vi "BC Verify Minor Frame Subroutine.vi"(5 "Instruction ID":i32, 6 "Pointers":T1={"Major Command Pointer"=2206, "Major Data Pointer"=2206, "Minor Command Pointer"=2206, "Minor Data Pointer"=2206}, 7 "Target IC (1-8)":u8, 8 "error in (no error)":errorcluster, 11 "Bus Controller in":refnum<class "Bus Controller.lvclass">) -> (0 "error out":errorcluster, 3 "Bus Controller out":refnum<class "Bus Controller.lvclass">, 4 "Pointers out":T1={"Major Command Pointer"=2206, "Major Data Pointer"=2206, "Minor Command Pointer"=2206, "Minor Data Pointer"=2206})   [LabVIEW 2020, in "Unit Tests.lvlib" / "Bus Controller.lvclass"]
uses:
  Bus Controller.lvclass
  Data Pointers.ctl
  Frames & Messages/TypeDefs/BC Op Codes - Verbose.ctl
  Frames & Messages/TypeDefs/BC Condition Codes.ctl
  Bus Controller.lvclass/Bus Controller.ctl
  Dependencies/Registry/Registry.lvclass/Registry.ctl
  <vilib>/addons/_JKI Toolkits/Caraya/classes/Assert/Assert True.vi
  Dependencies/FPGA Interface/FPGA Interface.lvclass
  BCI-1553 API.lvlib
  <vilib>/addons/_JKI Toolkits/Caraya/classes/Assert/Assert.lvclass
  Dependencies/Registry/Registry.lvclass
  <vilib>/addons/_JKI Toolkits/Caraya/classes/Test/Test.lvclass
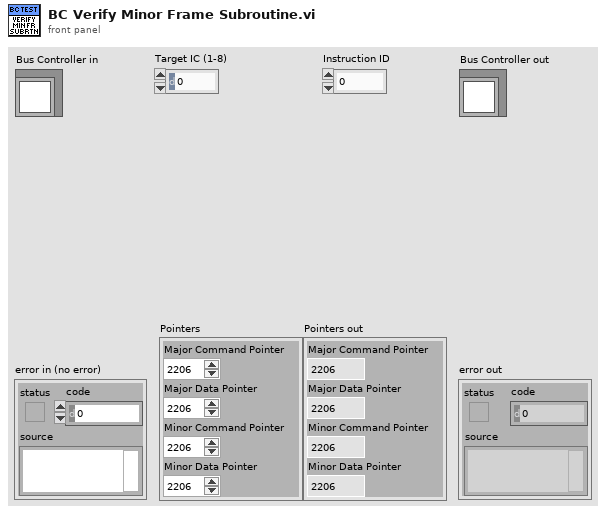
[diagram p1: front panel]
types:
  T1 = typedef "Data Pointers.ctl" = cluster{"Major Command Pointer":u16, "Major Data Pointer":u16, "Minor Command Pointer":u16, "Minor Data Pointer":u16}
  T2 = typedef "BCI-1553 API.lvlib/BC Condition Codes.ctl" = enum16{"GP0 == 1 || LT", "GP1 == 1 || NE", "GP2 == 1", "GP3 == 1", "GP4 == 1", "GP5 == 1", "GP6 == 1", "GP7 == 1", "NORESP", "FMTERR", "GOODBLOCK", "MSKSTATSET", "BADMSG", "1RETRY", "2RETRY", "ALWAYS"}
  T3 = typedef "BCI-1553 API.lvlib/BC Op Codes - Verbose.ctl" = enum16{"EXECUTE MSG", "EXECUTE MSG GO", "JUMP", "CALL SUBROUTINE", "RETURN", "INTERRUPT REQUEST", "HALT", "DELAY", "WAIT FRAME TIMER = 0", "COMPARE FRAME TIMER", "COMPARE MSG TIMER", "LOAD TIME TAG CTR", "LOAD TIME TAG CTR HI", "LOAD FRAME TIMER", "START FRAME TIMER", "PUSH TIME TAG COUNT", "PUSH TIME TAG COUNT HI", "PUSH TIME TAG COUNT BOTH", "PUSH BLOCK STATUS WORD", "PUSH CURRENT VALUE", "PUSH INDIRECT", "WAIT EXT TRIGGER", "EXECUTE AND FLIP", "EXECUTE, FLIP, GO", "WRITE VALUE TO WMI", "WRITE VALUE TO MEM", "DECREMENT RAM, SKIP", "FLAG"}
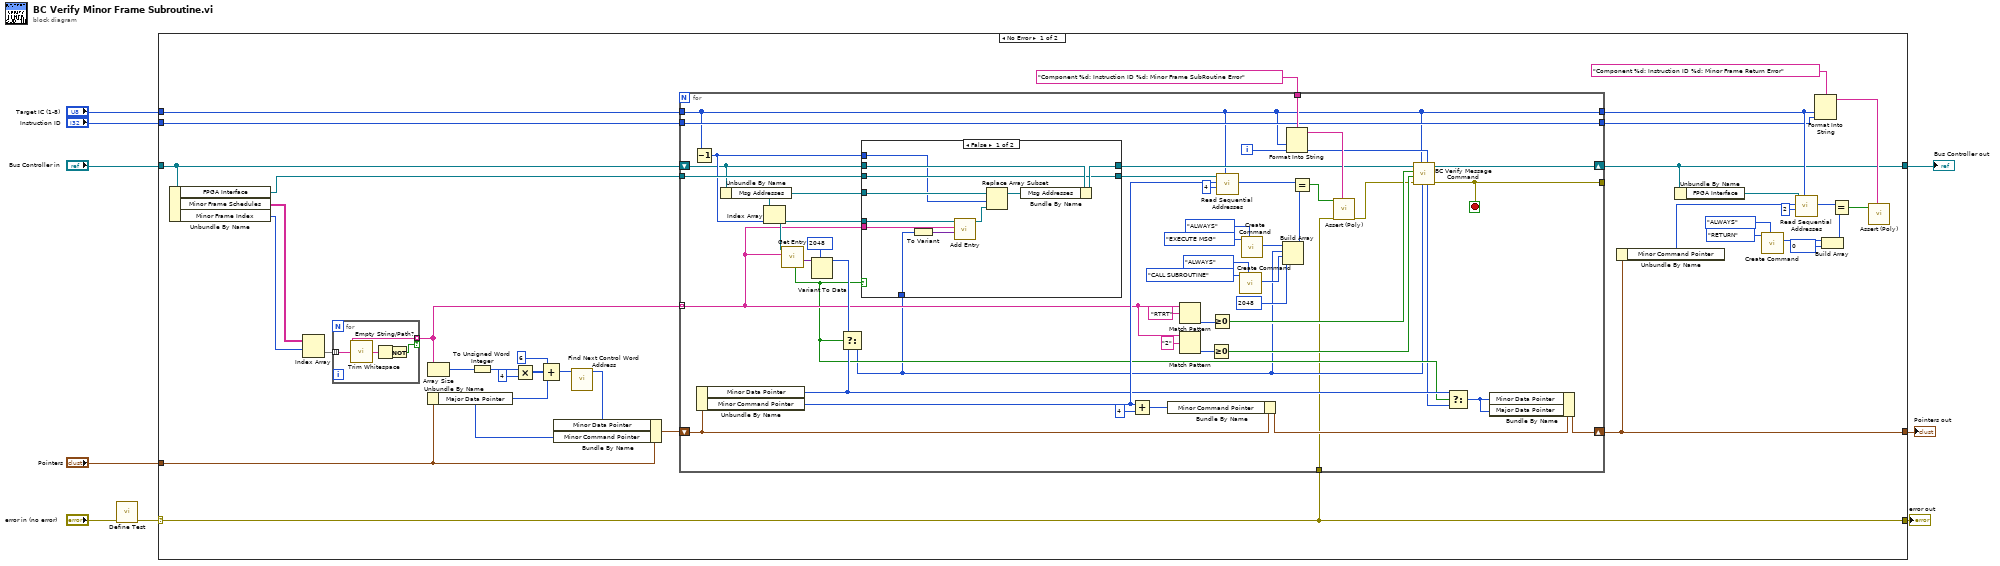
[diagram p0: block diagram]
diagram:
  n1 = call <vilib>:"Define Test.vi"("error in (no error)"="error in (no error)") -> ("error out"=w1:errorcluster)  [unwired: 9 in, 1 out]
  n2 = case shown="No Error" w1 {
    selector: w1 -> [w10 w112]
    tunnel: [w10 w112] -> w9
    tunnel: [w12 w111] -> w7
    tunnel: "Bus Controller in" -> [w31 w111]
    tunnel: "Pointers" -> [w32 _]
    tunnel: "Target IC (1-8)" -> [w29 _]
    tunnel: "Instruction ID" -> [w28 _]
    tunnel: [w11 _] -> w3
    frame No Error {
      n3 = Unbundle By Name(w31) -> ("FPGA Interface"=w30:refnum<class "FPGA Interface.lvclass">, "Minor Frame Schedules"=w35:string[][], "Minor Frame Index"=w36:i32)
      n4 = Index Array(array=w35, index (row)=w36) -> (element=w40:string[])  [unwired: 1 in]
      n5 = for {
        tunnel: w40 -> [w109] mode=indexing
        tunnel: [w109] -> w34 mode=indexing if=w107
        n6 = call <vilib>:"Trim Whitespace.vi"("string"=w109) -> ("trimmed string"=w110:string)  [unwired: 1 in]
        n7 = Empty String/Path?(string/path=w110) -> (empty?=w108:bool)
        n8 = Not(x=w108) -> (.not. x?=w107:bool)
      }
      n9 = Array Size(array=w34) -> (size(s)=w39:i32)
      n10 = Unbundle By Name(w32) -> ("Major Data Pointer"=w37:u16)
      n11 = To Unsigned Word Integer(number=w39) -> (unsigned 16bit integer=w41:u16)
      n12 = Multiply(x=w41, y=u16 4) -> (x*y=w43:u16)
      n13 = Compound Arithmetic op=ADD(u16 6 ("value"), w43, w37) -> (w45:u16)
      n14 = call "Find Next Control Word Address.vi"("Starting Address"=w45) -> ("0xHHHX Address"=w38:u16)  [unwired: 10 in]
      n15 = Bundle By Name(cluster=w32, "Minor Data Pointer"=w38, "Minor Command Pointer"=w37) -> (w33:T1)
      n16 = for {
        tunnel: [w54] -> _
        tunnel: w34 -> [w59] mode=indexing
        tunnel: "Component %d: Instruction ID %d: Minor Frame SubRoutine Error" ("message (\"\")") -> [w91]
        tunnel: w29 -> [w48]
        tunnel: w28 -> [w77]
        tunnel: w30 -> [w73]
        tunnel: [w48] -> w16
        tunnel: [w77] -> w15
        shift-right: [w69] -> w11
        shift-left: w33 -> [w66]
        shift-right: [w55] -> w12
        shift-left: w31 -> [w61]
        tunnel: w10 -> [w46]
        i -> [w49]
        stop <- w54 stop-if-true
        n17 = Decrement(x=w48) -> (x-1=w71:u8)
        n18 = Unbundle By Name(w66) -> ("Minor Data Pointer"=w68:u16, "Minor Command Pointer"=w70:u16)
        n19 = Unbundle By Name(w61) -> ("Msg Addresses"=w72:refnum<class "Registry.lvclass">[])
        n20 = Index Array(array=w72, index=w71) -> (element=w60:refnum<class "Registry.lvclass">)
        n21 = call "Get Entry.vi"("Key"=w59, "Registry in"=w60) -> ("Value"=w57:variant, "Found?"=w58:bool)  [unwired: 6 in, 2 out]
        n22 = Variant To Data(type=u16 2048, Variant=w57) -> (data=w75:u16)  [unwired: 1 in, 1 out]
        n23 = Select(t=w75, s=w58, f=w68) -> (s? t:f=w50:u16)
        n24 = case shown="False" w58 {
          tunnel: w59 -> [w96 _]
          tunnel: w50 -> [w104 _]
          tunnel: [w101 w106] -> w74
          tunnel: w73 -> [w101 w106]
          tunnel: [w102 w105] -> w56
          tunnel: w61 -> [w103 w105]
          tunnel: w71 -> [w98 _]
          tunnel: w60 -> [w97 _]
          tunnel: w72 -> [w100 _]
          frame False {
            n25 = To Variant(anything=w104) -> (Variant=w95:variant)
            n26 = call "Add Entry.vi"("Value"=w95, "Key"=w96, "Registry in"=w97) -> ("Registry out"=w94:refnum<class "Registry.lvclass">)  [unwired: 6 in, 2 out]
            n27 = Replace Array Subset(array=w100, new element=w94, index=w98) -> (w99:refnum<class "Registry.lvclass">[])
            n28 = Bundle By Name(cluster=w103, "Msg Addresses"=w99) -> (w102:refnum<class "Bus Controller.lvclass">)
          }
          frame True {
          }
        }
        n29 = Add(x=w70, y=u16 4) -> (x+y=w67:u16)
        n30 = Bundle By Name(cluster=w66, "Minor Command Pointer"=w67) -> (w65:T1)
        n31 = Match Pattern(string=w59, regular expression="RTRT") -> (offset past match=w81:i32)  [unwired: 1 in, 3 out]
        n32 = Match Pattern(string=w59, regular expression="2") -> (offset past match=w78:i32)  [unwired: 1 in, 3 out]
        n33 = Greater Or Equal To 0?(x=w78) -> (x >= 0?=w52:bool)
        n34 = Greater Or Equal To 0?(x=w81) -> (x >= 0?=w53:bool)
        n35 = call-dynamic "Read Sequential Addresses.vi"("Target IC (1-8)"=w48, "Addresses to Read"=u16 4, "Starting Address"=w70, "FPGA Interface in"=w74) -> ("Data"=w82:u16[])  [unwired: 6 in, 1 out]
        n36 = call "Create Command.vi"("Condition"=BC_Condition_Codes."ALWAYS", "Op Code"=BC_Op_Codes_-_Verbose."CALL SUBROUTINE") -> ("Instruction"=w86:u16)  [unwired: 8 in, 1 out]
        n37 = call "Create Command.vi"("Condition"=BC_Condition_Codes."ALWAYS", "Op Code"=BC_Op_Codes_-_Verbose."EXECUTE MSG") -> ("Instruction"=w85:u16)  [unwired: 8 in, 1 out]
        n38 = Build Array(w85, w50, w86, u16 2048) -> (w83:u16[])
        n39 = Format Into String(format string=w91, w48, w49) -> (resulting string=w62:string)  [unwired: 2 in, 1 out]
        n40 = Equal?(x=w82, y=w83) -> (x = y?=w63:bool)
        n41 = call-poly <vilib>:"Assert (Poly).vi"("Label"=w62, "error in (no error)"=w46, "True?"=w63) -> ("error out"=w47:errorcluster)  [unwired: 7 in, 1 out]
        n42 = call "BC Verify Message Command.vi"("Instruction ID"=w49, "Cmd Address"=w50, "Target IC (1-8)"=w48, "error in (no error)"=w47, "Transmit?"=w52, "RT-RT?"=w53, "Bus Controller in"=w56) -> ("error out"=w54:errorcluster, "Bus Controller out"=w55:refnum<class "Bus Controller.lvclass">, "Post-Data Address"=w51:u16)  [unwired: 2 in]
        n43 = Select(t=w68, s=w58, f=w51) -> (s? t:f=w64:u16)
        n44 = Bundle By Name(cluster=w65, "Minor Data Pointer"=w64, "Major Data Pointer"=w64) -> (w69:T1)
      }
      n45 = Unbundle By Name(w11) -> ("Minor Command Pointer"=w19:u16)
      n46 = Unbundle By Name(w12) -> ("FPGA Interface"=w18:refnum<class "FPGA Interface.lvclass">)
      n47 = call "Create Command.vi"("Condition"=BC_Condition_Codes."ALWAYS", "Op Code"=BC_Op_Codes_-_Verbose."RETURN") -> ("Instruction"=w23:u16)  [unwired: 8 in, 1 out]
      n48 = call-dynamic "Read Sequential Addresses.vi"("Target IC (1-8)"=w16, "Addresses to Read"=u16 2, "Starting Address"=w19, "FPGA Interface in"=w18) -> ("Data"=w26:u16[])  [unwired: 6 in, 1 out]
      n49 = Format Into String(format string="Component %d: Instruction ID %d: Minor Frame Return Error" ("message (\"\")"), w16, w15) -> (resulting string=w13:string)  [unwired: 2 in, 1 out]
      n50 = Build Array(w23, u16 0 ("element")) -> (w20:u16[])
      n51 = Equal?(x=w26, y=w20) -> (x = y?=w14:bool)
      n52 = call-poly <vilib>:"Assert (Poly).vi"("Label"=w13, "True?"=w14) -> ()  [unwired: 8 in, 2 out]
    }
    frame Error {
    }
  }
  "error out" <- w9
  "Bus Controller out" <- w7
  "Pointers out" <- w3
